vi "ex6-1.vi"   [LabVIEW 2013]
uses:
  <vilib>/NXT/Dual Mode Library/Waits/Wait_Touch.vi
  <vilib>/NXT/NXTIO Xnodes/NXTIONodeSubVIs/LEGOMoveAllMotors.vi
  <vilib>/NXT/NXTIO Xnodes/NXTIONodeSubVIs/LEGOStopAllMotors.vi
  <vilib>/NXT/Subs/LVHSConnector.ctl
  <vilib>/NXT/NXTIO Xnodes/NXTIOXNode/NXTIO.xnode
  <vilib>/NXT/LegoClasses/BrickReference/BrickReference.lvclass
types:
  T1 = typedef "LVHSConnector.ctl" = refnum<class "BrickReference.lvclass">
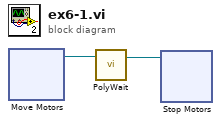
[diagram p0: block diagram]
diagram:
  n1 = xnode "Move Motors"() -> ("NXT/EV3"=w2:T1)  [unwired: 3 in]
  n2 = call-poly <vilib>:"PolyWait.vi"("NXT/EV3"=w2) -> ("NXT/EV3"=w1:T1)  [unwired: 3 in]
  n3 = xnode "Stop Motors"("NXT/EV3"=w1) -> ()  [unwired: 1 in, 1 out]
